vi "New Event Handler.vi"() -> ()   [LabVIEW 2010]
doc: "Compare this VI to the Old Event Handler.vi in this LLB. This VI uses Event structures to determine how to handle events instead of using polling. It is easier to understand how transitions work between different cases and requires just one shift register to maintain the data passed between different events. It does not poll the user interface to determine when a button is clicked but instead it waits for events like button clicks and value changes to occur and then decides what to do based on which event occured.\n\n\"Acquire Data\":\nClicking this button executes the case that acquires data. \n\n\"Analyze and Present Data\":\nClicking this button analyzes the data previously acquired. It is not necessary to acquire any data before clicking this button, but analysis done to a NULL dataset does not provide any useful information.\n\n\"Stop\":\nClicking this button stops the execution of the VI."
panel:
  in  "New Button":bool
  in  "Time Waveform":waveform(dbl)={"t0"=timestamp(0 s since 1904-01-01), "dt"=0.0, "Y"=[]}
  in  "Stop":bool
  in  "Analyze":bool
  in  "Acquire":bool
  # "Run the VI, and then press the\nbuttons to activate the corresponding\nevents.  Press the Stop button when\nfinished."
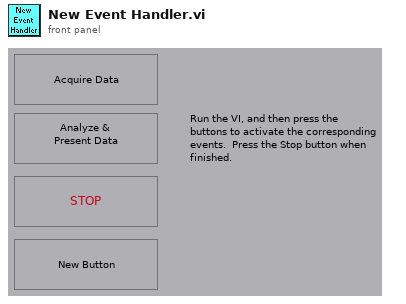
[diagram p1: front panel]
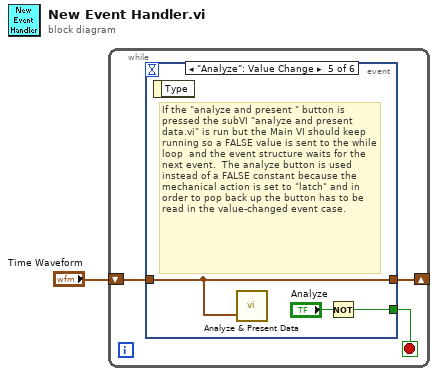
[diagram p0: block diagram]
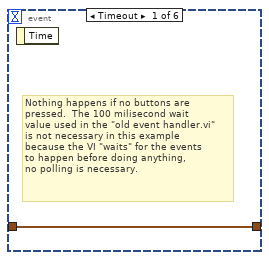
[diagram p2: hidden frame]
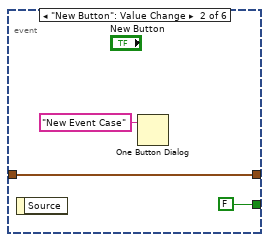
[diagram p3: hidden frame]
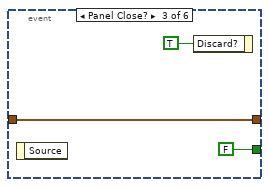
[diagram p4: hidden frame]
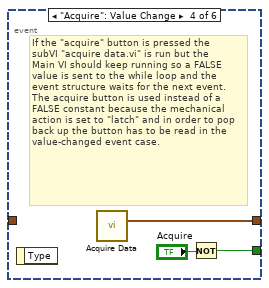
[diagram p5: hidden frame]
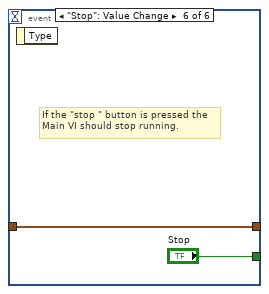
[diagram p6: hidden frame]
diagram:
  n1 = while {
    shift-right: [w4] -> _
    shift-left: "Time Waveform" -> [w3]
    stop <- w2 stop-if-true
    n2 = event shown="[4] \"Analyze\": Value Change" {
      selector: _ -> [_ _ _ _ _ _]
      dyn-events: _ -> [_ _ _ _ _ _]
      timeout: _ -> [_ _ _ _ _ _]
      tunnel: [w5 w8 w10 w14 w17 w19] -> w4
      tunnel: w3 -> [w5 w8 w10 _ w17 w19]
      tunnel: [_ FALSE ("Stop") FALSE ("Stop") w12 w15 "Stop"] -> w2
      event Timeout {
        # "Nothing happens if no buttons are \npressed.  The 100 milisecond wait \nvalue used in the \"old event handler.vi\" \nis not necessary in this example \nbecause the VI \"waits\" for the events \nto happen before doing anything, \nno polling is necessary."
        n3 = event-data() -> ()  [unwired: 1 in, 1 out]
      }
      event "New Button": Value Change {
        n4 = event-data() -> ()  [unwired: 1 in, 1 out]
        n5 = One Button Dialog(message="New Event Case") -> ()  [unwired: 1 in, 1 out]
      }
      event Panel Close? {
        n6 = event-data() -> ()  [unwired: 1 in, 1 out]
        n7 = event-data("Discard?"=TRUE) -> ()  [unwired: 1 in, 1 out]
      }
      event "Acquire": Value Change {
        # "If the \"acquire\" button is pressed the \nsubVI \"acquire data.vi\" is run but the\nMain VI should keep running so a FALSE value is sent to the while loop and the event structure waits for the next event.\nThe acquire button is used instead of a FALSE constant because the mechanical action is set to \"latch\" and in order to pop back up the button has to be read in the value-changed event case."
        n8 = event-data() -> ()  [unwired: 1 in, 1 out]
        n9 = call "Acquire Data.vi"() -> ("Time Waveform"=w14:waveform(dbl))  [unwired: 2 in]
        n10 = Not(x="Acquire") -> (.not. x?=w12:bool)
      }
      event "Analyze": Value Change {
        # "If the \"analyze and present \" button is \npressed the subVI \"analyze and present data.vi\" is run but the Main VI should keep running so a FALSE value is sent to the while loop  and the event structure waits for the next event.  The analyze button is used instead of a FALSE constant because the mechanical action is set to \"latch\" and in order to pop back up the button has to be read in the value-changed event case."
        n11 = event-data() -> ()  [unwired: 1 in, 1 out]
        n12 = call "Analyze & Present Data.vi"("Data"=w17) -> ()  [unwired: 2 in]
        n13 = Not(x="Analyze") -> (.not. x?=w15:bool)
      }
      event "Stop": Value Change {
        # "If the \"stop \" button is pressed the\nMain VI should stop running."
        n14 = event-data() -> ()  [unwired: 1 in, 1 out]
      }
    }
  }
